vi "DualEncoder.vi"(8 "error in (no error)":errorcluster, 11 "Reset?":bool) -> (0 "error out":errorcluster, 1 "Distance Right (in)":dbl, 2 "Distance Left (in)":dbl, 3 "Total Distance (in)":dbl)   [LabVIEW 2012]
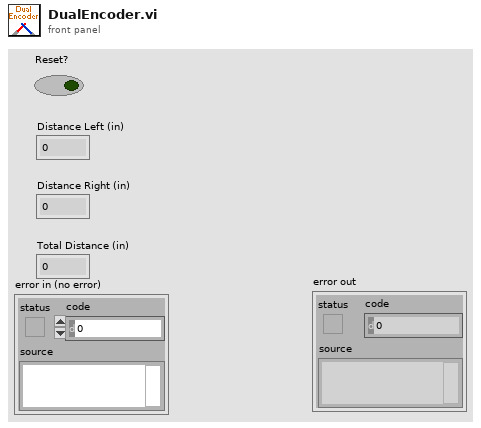
[diagram p1: front panel]
types:
  T1 = typedef "WPI_EncoderDevRef.ctl" = cluster{"DevStatus":errorcluster, "EncoderIndex":T2, "CounterIndex":T3, "DistancePerCount":dbl, "Decoding Type":T4}
  T2 = typedef "FPGA_EncoderIdx.ctl" = enum8{"Enc 0", "Enc 1", "Enc 2", "Enc 3", "Invalid"}
  T3 = typedef "FPGA_CounterCtrSystemIndex.ctl" = enum8{"Ctr 0", "Ctr 1", "Ctr 2", "Ctr 3", "Ctr 4", "Ctr 5", "Ctr 6", "Ctr 7", "Invalid"}
  T4 = typedef "WPI_EncoderType.ctl" = enum16{"1x", "2x", "4x"}
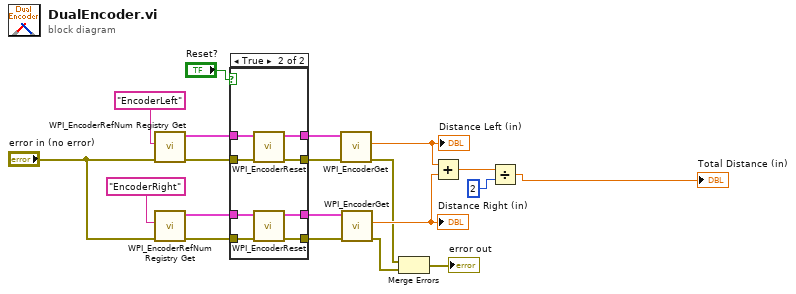
[diagram p0: block diagram]
diagram:
  n1 = call <vilib>:"WPI_EncoderRefNum Registry Get.vi"("error in (no error)"="error in (no error)", "refnum name"="EncoderLeft") -> ("error out"=w14:errorcluster, "EncoderDevRef"=w15:T1)  [unwired: 8 in]
  n2 = call <vilib>:"WPI_EncoderRefNum Registry Get.vi"("error in (no error)"="error in (no error)", "refnum name"="EncoderRight") -> ("error out"=w16:errorcluster, "EncoderDevRef"=w17:T1)  [unwired: 8 in]
  n3 = case shown="True" "Reset?" {
    tunnel: w17 -> [w22 w32]
    tunnel: w16 -> [w21 w31]
    tunnel: w15 -> [w24 w30]
    tunnel: w14 -> [w23 w29]
    tunnel: [w24 w28] -> w12
    tunnel: [w23 w27] -> w11
    tunnel: [w22 w26] -> w10
    tunnel: [w21 w25] -> w9
    frame False {
    }
    frame True {
      n4 = call <vilib>:"WPI_EncoderReset.vi"("error in (no error)"=w29, "EncoderDevRef"=w30) -> ("error out"=w27:errorcluster, "EncoderDevRef"=w28:T1)  [unwired: 8 in]
      n5 = call <vilib>:"WPI_EncoderReset.vi"("error in (no error)"=w31, "EncoderDevRef"=w32) -> ("error out"=w25:errorcluster, "EncoderDevRef"=w26:T1)  [unwired: 8 in]
    }
  }
  n6 = call <vilib>:"WPI_EncoderGet.vi"("error in (no error)"=w11, "EncoderDevRef"=w12) -> ("error out"=w4:errorcluster, "Distance"=w2:dbl)  [unwired: 4 in, 4 out]
  "Distance Left (in)" <- w2
  n7 = call <vilib>:"WPI_EncoderGet.vi"("error in (no error)"=w9, "EncoderDevRef"=w10) -> ("error out"=w3:errorcluster, "Distance"=w6:dbl)  [unwired: 4 in, 4 out]
  "Distance Right (in)" <- w6
  n8 = Merge Errors(w4, w3) -> (→"error out":errorcluster)
  n9 = Add(x=w2, y=w6) -> (x+y=w7:dbl)
  n10 = Divide(x=w7, y=2) -> (x/y=→"Total Distance (in)":dbl)
